vi "launch.vi"() -> ()   [LabVIEW 2017]
panel:
  out "字符串":string
  out "新版本号":string
  out "版本路径":path
  out "是否调用":bool=TRUE
  out "下载路径":string
  out "消息框":string
  # "请以管理员身份运行"
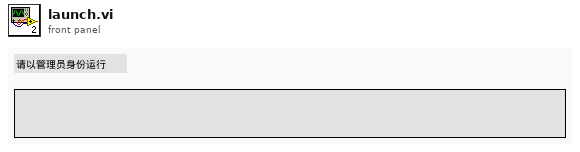
[diagram p1: front panel]
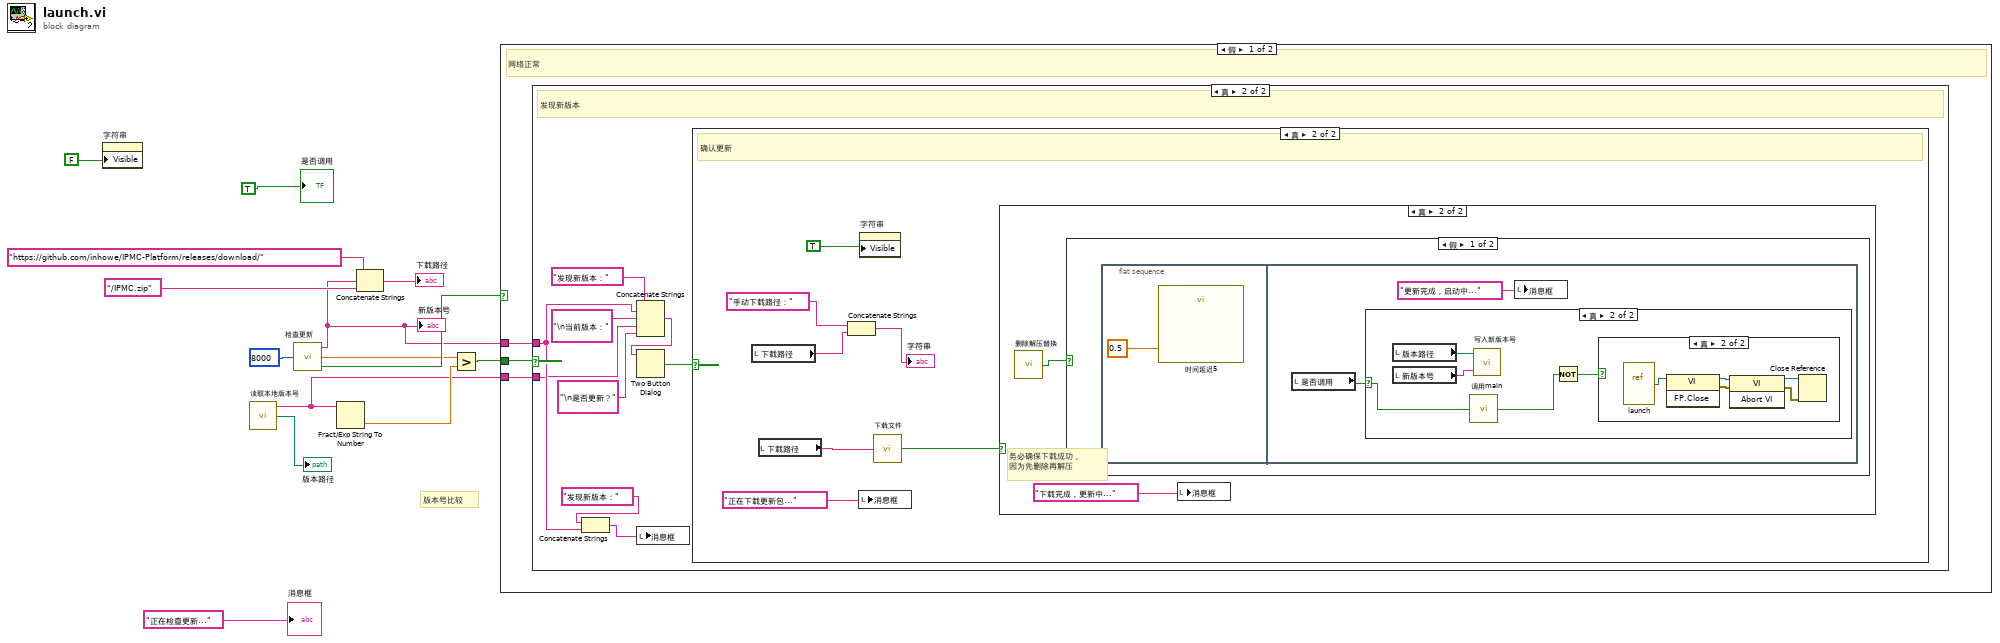
[diagram p0: block diagram]
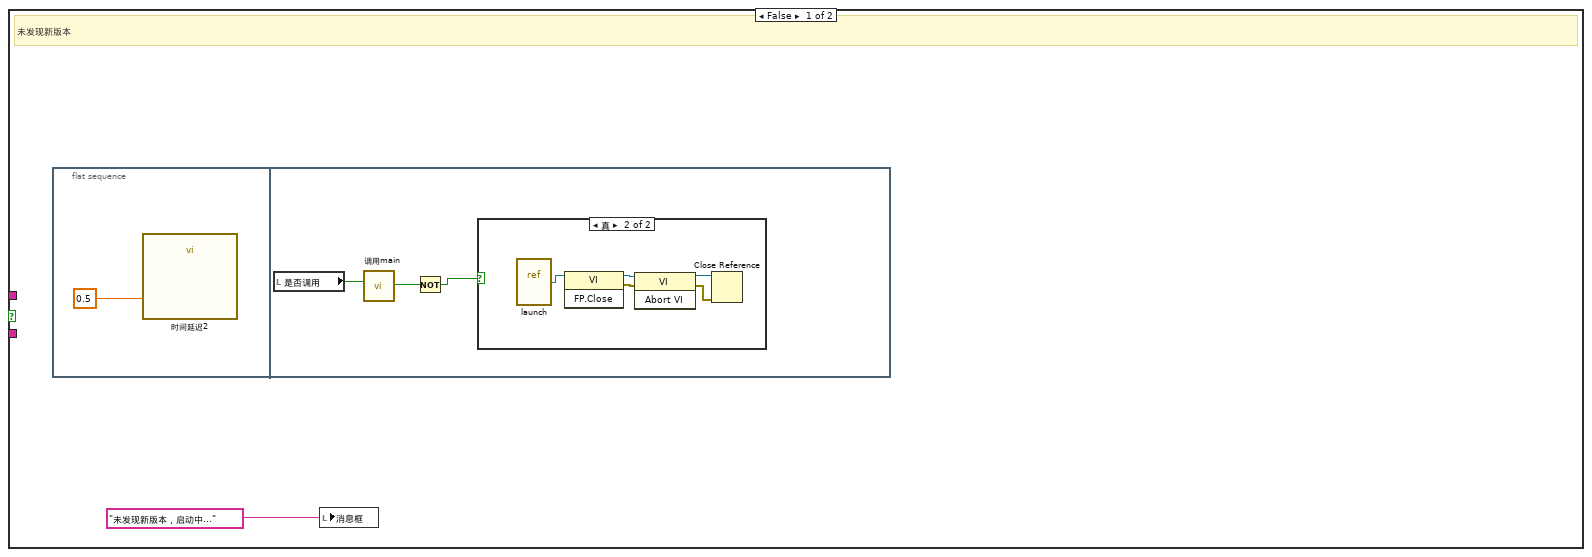
[diagram p2: hidden frame]
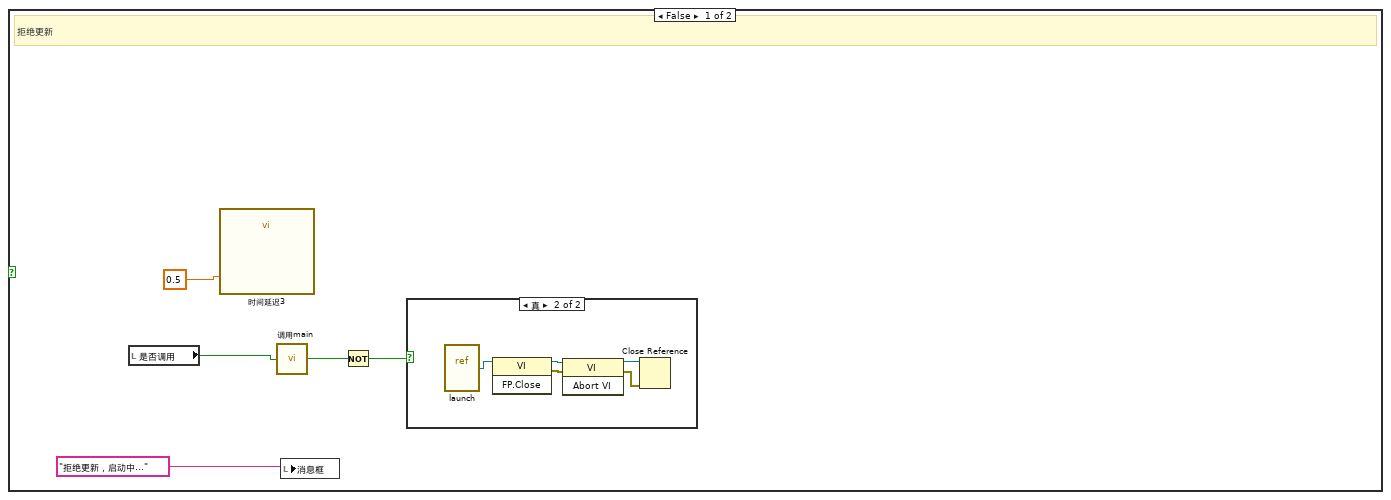
[diagram p4: hidden frame]
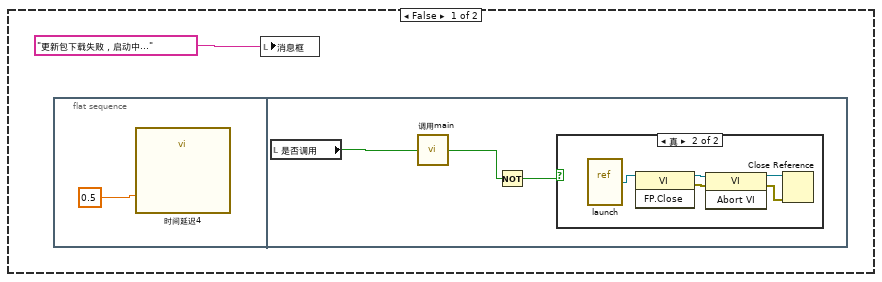
[diagram p6: hidden frame]
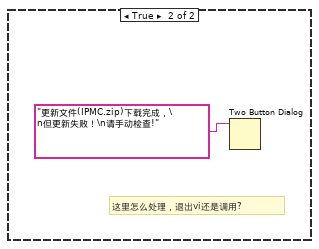
[diagram p10: hidden frame]
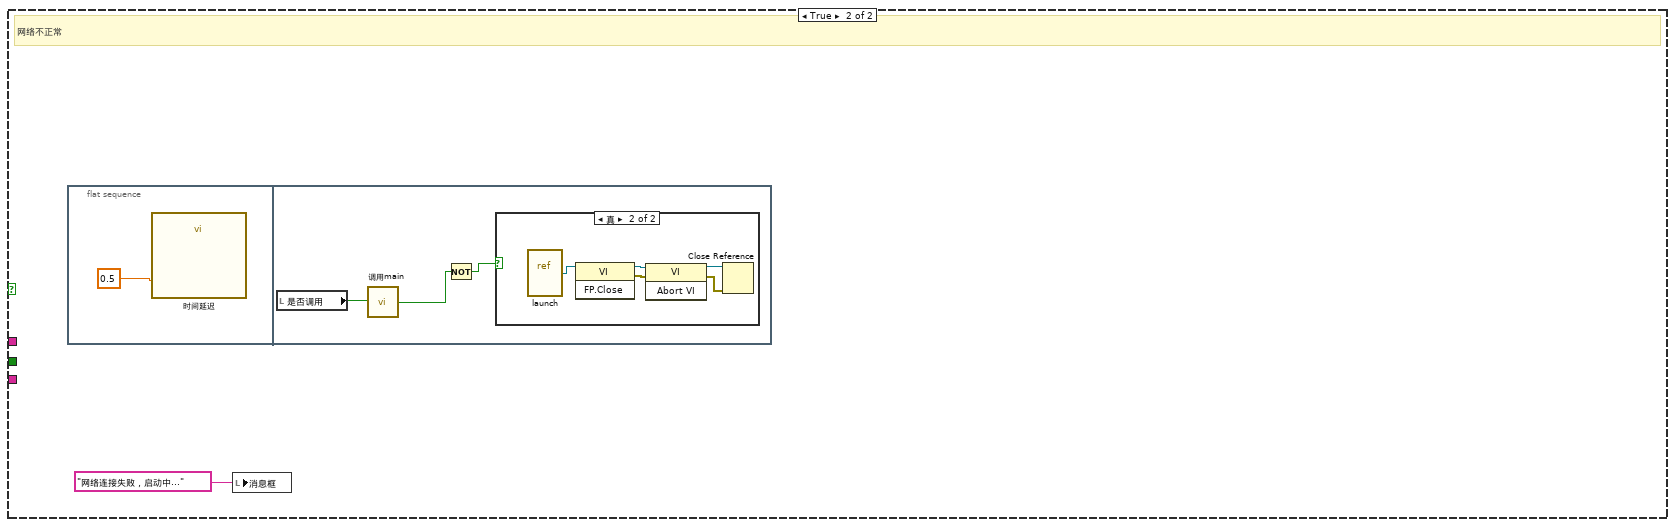
[diagram p11: hidden frame]
diagram:
  # "版本号比较"
  n1 = property on="字符串" class="Str"("Visible"=FALSE) -> ()  [unwired: 2 in, 2 out]
  n2 = call "读取本地版本号.vi"() -> ("版本号"=w1:string, "版本路径"=→"版本路径":path)  [unwired: 6 in, 1 out]
  n3 = call "检查更新.vi"("超时ms"=8000) -> (1:"新版本号"=w2:string, 2:"新版本号"=w5:dbl, "错误?"=w14:bool)
  "新版本号" <- w2
  n4 = Fract/Exp String To Number(string=w1) -> (number=w4:dbl)  [unwired: 3 in, 1 out]
  n5 = Concatenate Strings("https://github.com/inhowe/IPMC-Platform/releases/download/", w2, "/IPMC.zip") -> (→"下载路径":string)
  n6 = Greater?(x=w5, y=w4) -> (0:w11:bool)
  n7 = case "条件结构" shown="假" w14 {
    tunnel: w11 -> [w17 _]
    tunnel: w2 -> [w16 _]
    tunnel: w1 -> [w15 _]
    frame False {
      # "网络正常"
      n8 = case "条件结构" shown="真" w17 {
        tunnel: w16 -> [_ w32]
        tunnel: w15 -> [_ w29]
        frame False {
          # "未发现新版本"
          n9 = flat-sequence {
            frame #0 {
              n10 = call "时间延迟2"("Delay Time (s)"=0.5) -> ()  [unwired: 10 in, 1 out]
            }
            frame #1 {
              n11 = local read "是否调用"() -> (w22:bool)
              n12 = call "调用main.vi"("是否调用?"=w22) -> ("发生错误?"=w20:bool)
              n13 = Not(x=w20) -> (.not. x?=w21:bool)
              n14 = case shown="真" w21 {
                frame False {
                }
                frame True {
                  n15 = vi-ref "launch.vi"() -> (w27:refnum<vi>)
                  n16 = invoke class="VI" method="FP.Close"(reference=w27) -> (reference out=w26:refnum<vi>, error out=w25:errorcluster)  [unwired: 2 in, 1 out]
                  n17 = invoke class="VI" method="Abort VI"(reference=w26, error in=w25) -> (reference out=w24:refnum<vi>, error out=w23:errorcluster)  [unwired: 1 in, 1 out]
                  n18 = Close Reference(reference=w24, error in (no error)=w23) -> ()  [unwired: 1 out]
                }
              }
            }
          }
          n19 = local write "消息框"("未发现新版本，启动中...") -> ()
        }
        frame True {
          # "发现新版本"
          n20 = Concatenate Strings("发现新版本：", w32) -> (w31:string)
          n21 = Concatenate Strings("发现新版本：", w32, "\n当前版本：", w29, "\n是否更新？") -> (w34:string)
          n22 = Two Button Dialog(message=w34) -> (T button?=w36:bool)  [unwired: 2 in]
          n23 = local write "消息框"(w31) -> ()
          n24 = case "条件结构" shown="真" w36 {
            frame False {
              # "拒绝更新"
              n25 = local read "是否调用"() -> (w40:bool)
              n26 = call "时间延迟3"("Delay Time (s)"=0.5) -> ()  [unwired: 10 in, 1 out]
              n27 = call "调用main.vi"("是否调用?"=w40) -> ("发生错误?"=w38:bool)
              n28 = local write "消息框"("拒绝更新，启动中...") -> ()
              n29 = Not(x=w38) -> (.not. x?=w37:bool)
              n30 = case shown="真" w37 {
                frame False {
                }
                frame True {
                  n31 = vi-ref "launch.vi"() -> (w46:refnum<vi>)
                  n32 = invoke class="VI" method="FP.Close"(reference=w46) -> (reference out=w45:refnum<vi>, error out=w44:errorcluster)  [unwired: 2 in, 1 out]
                  n33 = invoke class="VI" method="Abort VI"(reference=w45, error in=w44) -> (reference out=w43:refnum<vi>, error out=w42:errorcluster)  [unwired: 1 in, 1 out]
                  n34 = Close Reference(reference=w43, error in (no error)=w42) -> ()  [unwired: 1 out]
                }
              }
            }
            frame True {
              # "确认更新"
              n35 = local read "下载路径"() -> (w48:string)
              n36 = local read "下载路径"() -> (w52:string)
              n37 = Concatenate Strings("手动下载路径：", w48) -> (→"字符串":string)
              n38 = local write "消息框"("正在下载更新包...") -> ()
              n39 = property on="字符串" class="Str"("Visible"=TRUE) -> ()  [unwired: 2 in, 2 out]
              n40 = call "下载文件.vi"("URL"=w52) -> ("下载成功?"=w51:bool)
              n41 = case shown="真" w51 {
                frame False {
                  n42 = flat-sequence {
                    frame #0 {
                      n43 = call "时间延迟4"("Delay Time (s)"=0.5) -> ()  [unwired: 10 in, 1 out]
                    }
                    frame #1 {
                      n44 = local read "是否调用"() -> (w58:bool)
                      n45 = call "调用main.vi"("是否调用?"=w58) -> ("发生错误?"=w56:bool)
                      n46 = Not(x=w56) -> (.not. x?=w57:bool)
                      n47 = case shown="真" w57 {
                        frame False {
                        }
                        frame True {
                          n48 = vi-ref "launch.vi"() -> (w63:refnum<vi>)
                          n49 = invoke class="VI" method="FP.Close"(reference=w63) -> (reference out=w62:refnum<vi>, error out=w61:errorcluster)  [unwired: 2 in, 1 out]
                          n50 = invoke class="VI" method="Abort VI"(reference=w62, error in=w61) -> (reference out=w60:refnum<vi>, error out=w59:errorcluster)  [unwired: 1 in, 1 out]
                          n51 = Close Reference(reference=w60, error in (no error)=w59) -> ()  [unwired: 1 out]
                        }
                      }
                    }
                  }
                  n52 = local write "消息框"("更新包下载失败，启动中...") -> ()
                }
                frame True {
                  # "务必确保下载成功，\n因为先删除再解压"
                  n53 = call "删除解压替换.vi"() -> ("操作失败?"=w65:bool)  [unwired: 1 in]
                  n54 = case shown="假" w65 {
                    frame False {
                      n55 = flat-sequence {
                        frame #0 {
                          n56 = call "时间延迟5"("Delay Time (s)"=0.5) -> ()  [unwired: 10 in, 1 out]
                        }
                        frame #1 {
                          n57 = local read "是否调用"() -> (w68:bool)
                          n58 = case shown="真" w68 {
                            selector: w68 -> [_ w71]
                            frame False {
                            }
                            frame True {
                              n59 = local read "版本路径"() -> (w72:path)
                              n60 = local read "新版本号"() -> (w73:string)
                              n61 = call "调用main.vi"("是否调用?"=w71) -> ("发生错误?"=w69:bool)
                              n62 = call "写入新版本号.vi"("版本路径(配置文件)"=w72, "版本号"=w73) -> ()  [unwired: 2 in, 1 out]
                              n63 = Not(x=w69) -> (.not. x?=w70:bool)
                              n64 = case shown="真" w70 {
                                frame False {
                                }
                                frame True {
                                n65 = vi-ref "launch.vi"() -> (w78:refnum<vi>)
                                n66 = invoke class="VI" method="FP.Close"(reference=w78) -> (reference out=w77:refnum<vi>, error out=w76:errorcluster)  [unwired: 2 in, 1 out]
                                n67 = invoke class="VI" method="Abort VI"(reference=w77, error in=w76) -> (reference out=w75:refnum<vi>, error out=w74:errorcluster)  [unwired: 1 in, 1 out]
                                n68 = Close Reference(reference=w75, error in (no error)=w74) -> ()  [unwired: 1 out]
                                }
                              }
                            }
                          }
                          n69 = local write "消息框"("更新完成，启动中...") -> ()
                        }
                      }
                    }
                    frame True {
                      # "这里怎么处理，退出vi还是调用?"
                      n70 = Two Button Dialog(message="更新文件(IPMC.zip)下载完成，\n但更新失败！\n请手动检查!") -> ()  [unwired: 2 in, 1 out]
                    }
                  }
                  n71 = local write "消息框"("下载完成，更新中...") -> ()
                }
              }
            }
          }
        }
      }
    }
    frame True {
      # "网络不正常"
      n72 = flat-sequence {
        frame #0 {
          n73 = call "时间延迟"("Delay Time (s)"=0.5) -> ()  [unwired: 10 in, 1 out]
        }
        frame #1 {
          n74 = local read "是否调用"() -> (w84:bool)
          n75 = call "调用main.vi"("是否调用?"=w84) -> ("发生错误?"=w82:bool)
          n76 = Not(x=w82) -> (.not. x?=w83:bool)
          n77 = case shown="真" w83 {
            frame False {
            }
            frame True {
              n78 = vi-ref "launch.vi"() -> (w89:refnum<vi>)
              n79 = invoke class="VI" method="FP.Close"(reference=w89) -> (reference out=w88:refnum<vi>, error out=w87:errorcluster)  [unwired: 2 in, 1 out]
              n80 = invoke class="VI" method="Abort VI"(reference=w88, error in=w87) -> (reference out=w86:refnum<vi>, error out=w85:errorcluster)  [unwired: 1 in, 1 out]
              n81 = Close Reference(reference=w86, error in (no error)=w85) -> ()  [unwired: 1 out]
            }
          }
        }
      }
      n82 = local write "消息框"("网络连接失败，启动中...") -> ()
    }
  }
  "消息框" <- "正在检查更新..."
  "是否调用" <- TRUE
